vi "Config Display UI.vi"(8 "error in (no error)":errorcluster, 10 "Main Ctl and UI Ref":T1, 11 "Management in":refnum<class "Display.lvclass">) -> (0 "error out":errorcluster, 3 "Management out":refnum<class "Display.lvclass">)   [LabVIEW 2015, in "UserManagement.lvlib" / "Display.lvclass"]
uses:
  Display.lvclass
  typedef/Main Ctl and UI Ref.ctl
  Display.lvclass/Display.ctl
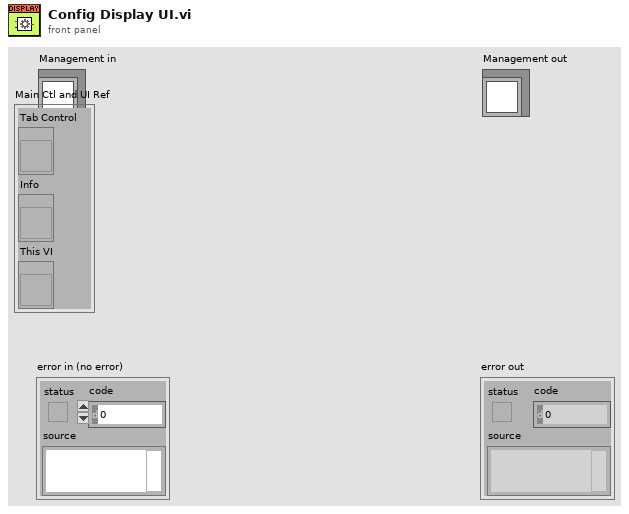
[diagram p1: front panel]
types:
  T1 = typedef "Main Ctl and UI Ref.ctl" = cluster{"Tab Control":refnum<vi>, "Info":refnum<vi>, "This VI":refnum<vi>}
  T2 = typedef "userOfLoginLaw.ctl" = enum16{"COMMONUSER", "ADMIN"}
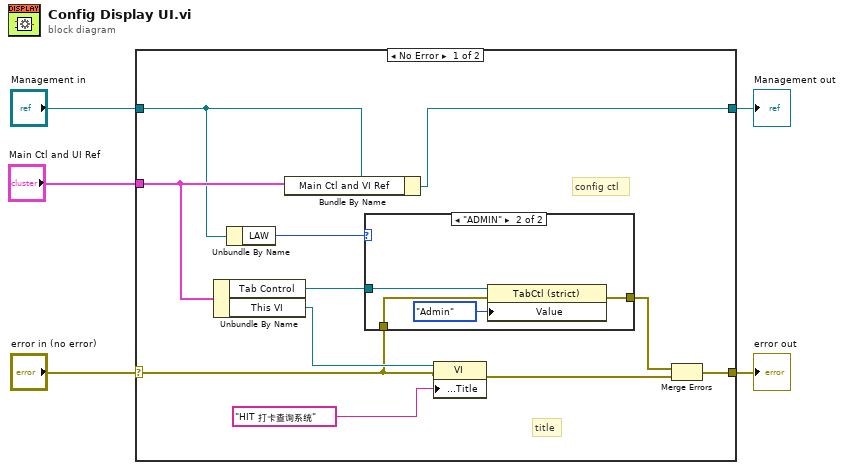
[diagram p0: block diagram]
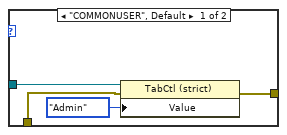
[diagram p2: hidden frame]
diagram:
  n1 = case shown="No Error" "error in (no error)" {
    selector: "error in (no error)" -> [w9 w26]
    tunnel: [w6 w26] -> w4
    tunnel: [w16 w25] -> w2
    tunnel: "Management in" -> [w14 w25]
    tunnel: "Main Ctl and UI Ref" -> [w15 _]
    frame No Error {
      # "title"
      # "config ctl"
      n2 = Unbundle By Name(w15) -> ("Tab Control"=w12:refnum<vi>, "This VI"=w11:refnum<vi>)
      n3 = Unbundle By Name(w14) -> ("LAW"=w13:T2)
      n4 = Bundle By Name(cluster=w14, "Main Ctl and VI Ref"=w15) -> (w16:refnum<class "Display.lvclass">)
      n5 = case shown="\"ADMIN\"" w13 {
        tunnel: w12 -> [w19 w24]
        tunnel: w9 -> [w17 w23]
        tunnel: [w18 w21] -> w8
        frame "COMMONUSER", Default {
          n6 = property class="TabCtl (strict)"(reference=w19, error in=w17, "Value"=enum32{"CommonUser", "Admin"}."Admin") -> (error out=w18:errorcluster)  [unwired: 1 out]
        }
        frame "ADMIN" {
          n7 = property class="TabCtl (strict)"(reference=w24, error in=w23, "Value"=enum32{"CommonUser", "Admin"}."Admin") -> (error out=w21:errorcluster)  [unwired: 1 out]
        }
      }
      n8 = property class="VI"(reference=w11, error in=w9, "Front Panel.Title"="HIT 打卡查询系统" ("Front Panel Window:Title")) -> (error out=w7:errorcluster)  [unwired: 1 out]
      n9 = Merge Errors(w8, w7) -> (w6:errorcluster)
    }
    frame Error {
    }
  }
  "error out" <- w4
  "Management out" <- w2
